vi "Populate Flat Cluster.vi"(7 "Prefix Name":string, 8 "error in (no error)":errorcluster, 9 "Values":string[](array[string]), 10 "Keys":string[](array[string]), 11 "Clust Refnum":refnum<vi>) -> (0 "error out":errorcluster, 3 "Cluster Refnum (Dup)":refnum<vi>)   [LabVIEW 2017]
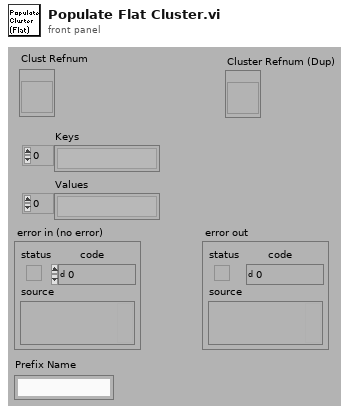
[diagram p1: front panel]
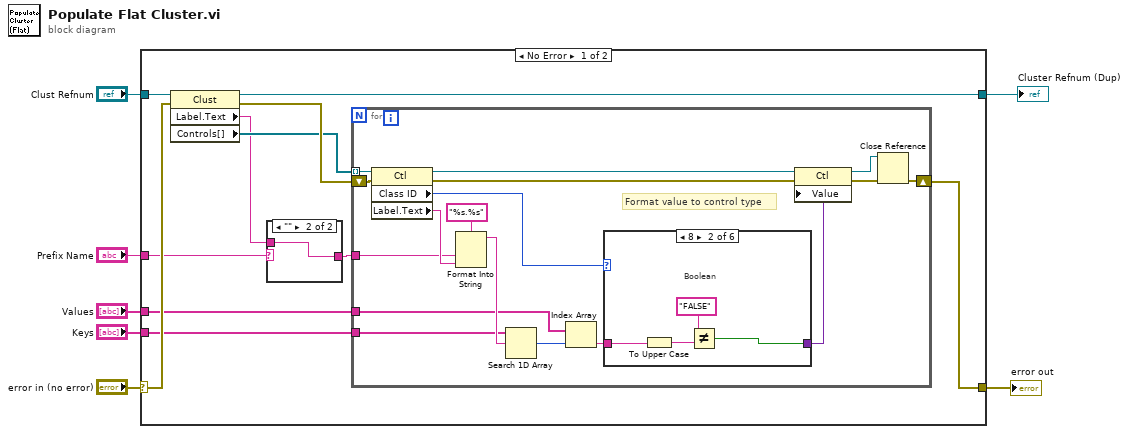
[diagram p0: block diagram]
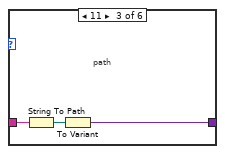
[diagram p4: hidden frame]
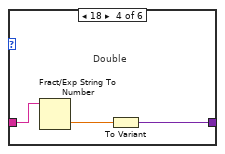
[diagram p5: hidden frame]
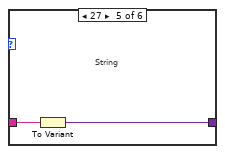
[diagram p6: hidden frame]
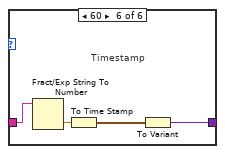
[diagram p7: hidden frame]
diagram:
  n1 = case shown="No Error" "error in (no error)" {
    selector: "error in (no error)" -> [w14 w54]
    tunnel: "Clust Refnum" -> [w16 w55]
    tunnel: [w15 w55] -> w6
    tunnel: [w13 w54] -> w5
    tunnel: "Prefix Name" -> [w10 _]
    tunnel: "Values" -> [w9 _]
    tunnel: "Keys" -> [w8 _]
    frame No Error {
      n2 = property class="Clust"(reference=w16, error in=w14) -> (reference out=w15:refnum<vi>, error out=w18:errorcluster, "Label.Text"=w11:string, "Controls[]"=w17:refnum<vi>[])
      n3 = case shown="\"\"" w10 {
        selector: w10 -> [w19 _]
        tunnel: [w19 w20] -> w12
        tunnel: w11 -> [_ w20]
        frame Default {
        }
        frame "" {
        }
      }
      n4 = for {
        tunnel: w17 -> [w37] mode=indexing
        tunnel: w8 -> [w26]
        tunnel: w9 -> [w27]
        shift-right: [w23] -> w13
        shift-left: w18 -> [w36]
        tunnel: w12 -> [w33]
        # "Format value to control type"
        n5 = property class="Ctl"(reference=w37, error in=w36) -> (reference out=w31:refnum<vi>, error out=w30:errorcluster, "Class ID"=w32:u32, "Label.Text"=w34:string)
        n6 = Format Into String(format string="%s.%s", w33, w34) -> (resulting string=w29:string)  [unwired: 2 in, 1 out]
        n7 = Search 1D Array(1D array=w26, element=w29) -> (index of element=w28:i32)  [unwired: 1 in]
        n8 = Index Array(array=w27, index=w28) -> (element=w21:string)
        n9 = case shown="8" w32 {
          tunnel: w21 -> [_ w41 w43 w47 w49 w53]
          tunnel: [_ w39 w44 w45 w48 w52] -> w22
          frame Default {
          }
          frame 8 {
            # "Boolean"
            n10 = To Upper Case(1:w41) -> (0:w38:string)
            n11 = Not Equal?(x="FALSE", y=w38) -> (x != y?=w39:bool)
          }
          frame 11 {
            # "path"
            n12 = String To Path(string=w43) -> (path=w42:path)
            n13 = To Variant(anything=w42) -> (Variant=w44:variant)
          }
          frame 18 {
            # "Double"
            n14 = Fract/Exp String To Number(string=w47) -> (number=w46:dbl)  [unwired: 3 in, 1 out]
            n15 = To Variant(anything=w46) -> (Variant=w45:variant)
          }
          frame 27 {
            # "String"
            n16 = To Variant(anything=w49) -> (Variant=w48:variant)
          }
          frame 60 {
            # "Timestamp"
            n17 = Fract/Exp String To Number(string=w53) -> (number=w51:dbl)  [unwired: 3 in, 1 out]
            n18 = To Time Stamp(1:w51) -> (0:w50:timestamp)
            n19 = To Variant(anything=w50) -> (Variant=w52:variant)
          }
        }
        n20 = property class="Ctl"(reference=w31, error in=w30, "Value"=w22) -> (reference out=w24:refnum<vi>, error out=w25:errorcluster)
        n21 = Close Reference(reference=w24, error in (no error)=w25) -> (error out=w23:errorcluster)
      }
    }
    frame Error {
    }
  }
  "error out" <- w5
  "Cluster Refnum (Dup)" <- w6
